vi "par_test.vi"() -> ()   [LabVIEW 2013]
uses:
  drivers/DMM/3458A Virtual Digitizer.lvlib
  drivers/DMM/3458A Virtual Channel Config.ctl
  drivers/Counter/Counter Type.ctl
  drivers/Counter/Counter.lvlib
  drivers/Counter/Counter Session.ctl
  drivers/AWG/AWG Type.ctl
  drivers/AWG/AWG.lvlib
  drivers/AWG/AWG Session.ctl
  drivers/DMM/3458A Sync Mode.ctl
  drivers/DMM/3458A Idn Mode.ctl
  drivers/DMM/3458A Data Packet.ctl
  drivers/DMM/3458A Digitizing Process Options.ctl
  drivers/DMM/3458A Digitizer Session.ctl
  drivers/DMM/3458A Aux Record Data.ctl
  drivers/DMM/3458A Digitizing Low Levels/Configure/Sampling Mode.ctl
  drivers/DMM/3458A Digitizing Low Levels/3458A Digitizing Low Levels.lvlib
panel:
  out "error out 6":errorcluster
  out "error out 5":errorcluster
  out "error out 4":errorcluster
  out "process exited 3":bool
  out "process exited 2":bool
  out "process exited":bool
  out "proc error out 3":errorcluster
  out "proc error out 2":errorcluster
  out "proc error out":errorcluster
  out "error out 3":errorcluster
  out "error out 2":errorcluster
  out "error out":errorcluster
  in  "digitizer session":T1 {"channels"."Range [Vpk]" min=0.0}
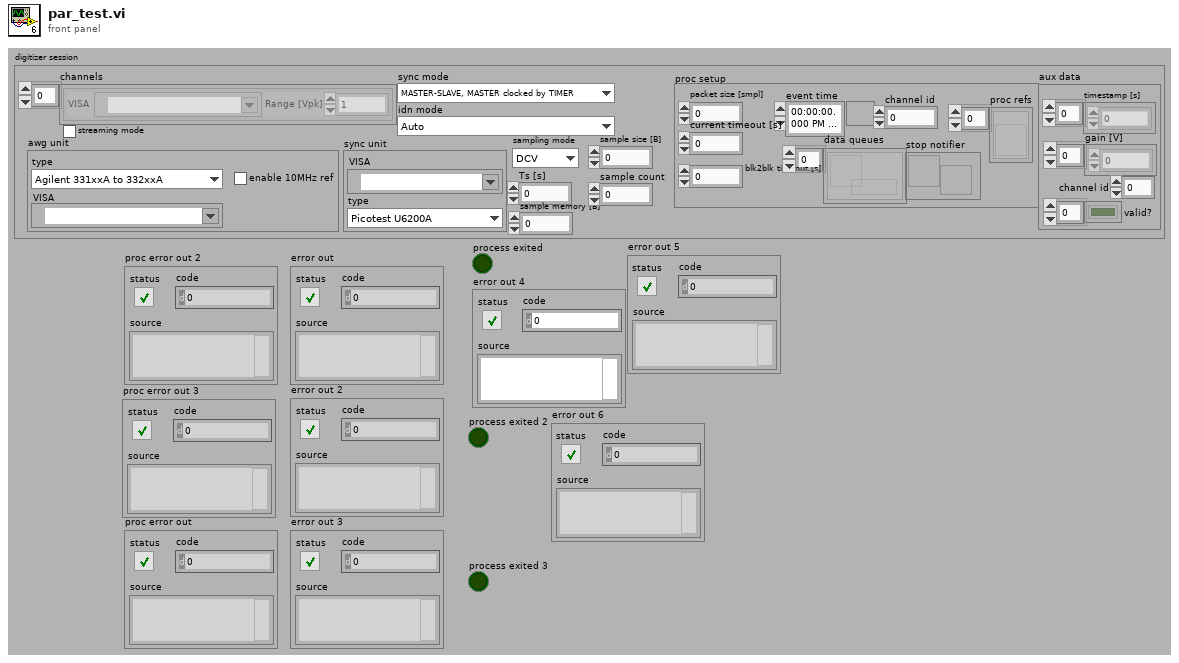
[diagram p1: front panel]
types:
  T1 = typedef "3458A Virtual Digitizer.lvlib/3458A Digitizer Session.ctl" = cluster{"channels":T2[], "sync unit":T3, "awg unit":T5, "sync mode":T7, "streaming mode":bool, "idn mode":T8, "sampling mode":T9, "Ts [s]":dbl, "sample memory [B]":i32, "proc setup":T10, "sample size [B]":i32, "sample count":i32, "aux data":T11}
  T2 = typedef "3458A Virtual Digitizer.lvlib/3458A Virtual Channel Config.ctl" = cluster{"VISA":refnum<visa-resource-name>, "Range [Vpk]":dbl}
  T3 = typedef "Counter.lvlib/Counter Session.ctl" = cluster{"VISA":refnum<visa-resource-name>, "type":T4}
  T4 = typedef "Counter.lvlib/Counter Type.ctl" = enum16{"Picotest U6200A", "dummy"}
  T5 = typedef "AWG.lvlib/AWG Session.ctl" = cluster{"type":T6, "VISA":refnum<visa-resource-name>, "enable 10MHz ref":bool}
  T6 = typedef "AWG.lvlib/AWG Type.ctl" = enum16{"Agilent 331xxA to 332xxA", "Agilent 335xxA to 336xxA", "dummy"}
  T7 = typedef "3458A Virtual Digitizer.lvlib/3458A Sync Mode.ctl" = enum16{"MASTER-SLAVE, MASTER clocked by TIMER", "MASTER-SLAVE, MASTER clocked by AWG", "ALL clocked by AWG", "MASTER-SLAVE, ALL clocked by TIMER", "ALL clocked by AWG with DFLL"}
  T8 = typedef "3458A Virtual Digitizer.lvlib/3458A Idn Mode.ctl" = enum16{"Auto", "Sequential (chn A, chn B, ...)", "From calibration string"}
  T9 = typedef "3458A Virtual Digitizer.lvlib/3458A Digitizing Low Levels.lvlib/Sampling Mode.ctl" = enum16{"DCV", "DSDC", "DSAC"}
  T10 = typedef "3458A Virtual Digitizer.lvlib/3458A Digitizing Process Options.ctl" = cluster{"channel id":i32, "packet size [smpl]":i32, "current timeout [s]":dbl, "blk2blk timeout [s]":dbl, "event time":timestamp, "stop notifier":refnum<notifier>, "data queues":refnum<queue>[], "proc refs":refnum<vi>[]}
  T11 = typedef "3458A Virtual Digitizer.lvlib/3458A Aux Record Data.ctl" = cluster{"channel id":i32, "valid?":bool[], "gain [V]":dbl[], "timestamp [s]":dbl[]}
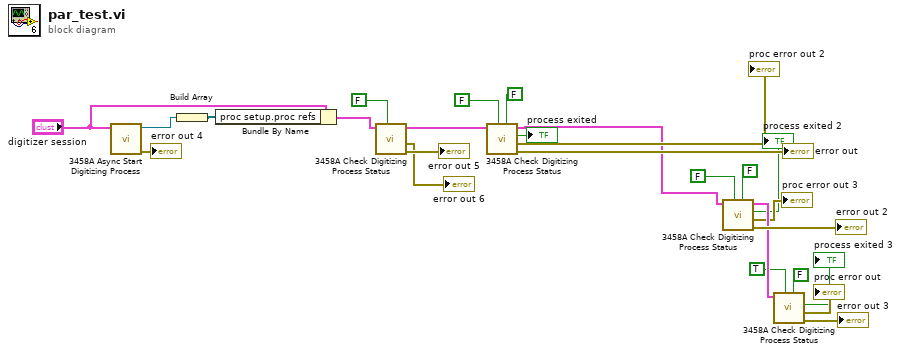
[diagram p0: block diagram]
diagram:
  n1 = call "3458A Async Start Digitizing Process.vi"("digitizer session"="digitizer session") -> ("error out"=→"error out 4":errorcluster, "vi ref out"=w24:refnum<vi>)  [unwired: 9 in]
  n2 = Build Array(w24) -> (w25:refnum<vi>[])
  n3 = Bundle By Name(cluster="digitizer session", "proc setup.proc refs"=w25) -> (w7:T1)
  n4 = call "3458A Check Digitizing Process Status.vi"("wait for exit (False)"=FALSE, "digitizer session in"=w7) -> ("error out"=→"error out 5":errorcluster, "proc error out"=→"error out 6":errorcluster, "digitizer session out"=w6:T1)  [unwired: 4 in, 3 out]
  n5 = call "3458A Check Digitizing Process Status.vi"("merge process exit error with main (True)"=FALSE, "wait for exit (False)"=FALSE, "digitizer session in"=w6) -> ("error out"=→"error out":errorcluster, "proc error out"=→"proc error out 2":errorcluster, "process exited?"=→"process exited":bool, "digitizer session out"=w3:T1)  [unwired: 3 in, 2 out]
  n6 = call "3458A Check Digitizing Process Status.vi"("merge process exit error with main (True)"=FALSE, "wait for exit (False)"=FALSE, "digitizer session in"=w3) -> ("error out"=→"error out 2":errorcluster, "proc error out"=→"proc error out 3":errorcluster, "process exited?"=→"process exited 2":bool, "digitizer session out"=w21:T1)  [unwired: 3 in, 2 out]
  n7 = call "3458A Check Digitizing Process Status.vi"("merge process exit error with main (True)"=FALSE, "wait for exit (False)"=TRUE, "digitizer session in"=w21) -> ("error out"=→"error out 3":errorcluster, "proc error out"=→"proc error out":errorcluster, "process exited?"=→"process exited 3":bool)  [unwired: 3 in, 3 out]
